vi "Quad PID 2015.vi"(0 "Target Velocity (rev/sec) 1":dbl, 1 "Measured Velocity (rev/sec) 1":dbl, 2 "Measured Velocity (rev/sec) 2":dbl, 3 "PID gains":T2 {"derivative time (Td, min)" format="%.3f"; "integral time (Ti, min)" format="%.3f"; "proportional gain (Kc)" format="%.3f"}, 5 "Target Velocity (rev/sec) 2":dbl, 9 "Target Velocity (rev/sec) 3":dbl, 11 "Target Velocity (rev/sec) 4":dbl, 12 "Measured Velocity (rev/sec) 3":dbl, 13 "Measured Velocity (rev/sec) 4":dbl, 14 "output range":cluster{"output high":dbl, "output low":dbl}={"output high"=1.0, "output low"=-1.0} {"output low" format="%.2f"; "output high" format="%.2f"}) -> (4 "Output Value (-1 to +1) 1":dbl format="%.2f", 6 "Output Value (-1 to +1) 2":dbl format="%.2f", 8 "Output Value (-1 to +1) 3":dbl format="%.2f", 10 "Output Value (-1 to +1) 4":dbl format="%.2f")   [LabVIEW 2014]
uses:
  <vilib>/Rock Robotics/WPI/DriverStation/WPI_DriverStationRobotMode2.ctl
  Robot Global Data.vi
  <vilib>/addons/control/pid/pid.llb/PID (DBL).vi
  <vilib>/addons/control/pid/NI_PID_pid.lvlib
panel:
  out "output cluster":T1(graph)
  in  "PID gains 2":T2={"proportional gain (Kc)"=2.0999999999999996, "integral time (Ti, min)"=0.004, "derivative time (Td, min)"=0.0} {"derivative time (Td, min)" format="%.3f"; "integral time (Ti, min)" min=0.0 step=0.001 format="%.3f"; "proportional gain (Kc)" step=0.05 format="%.3f"}
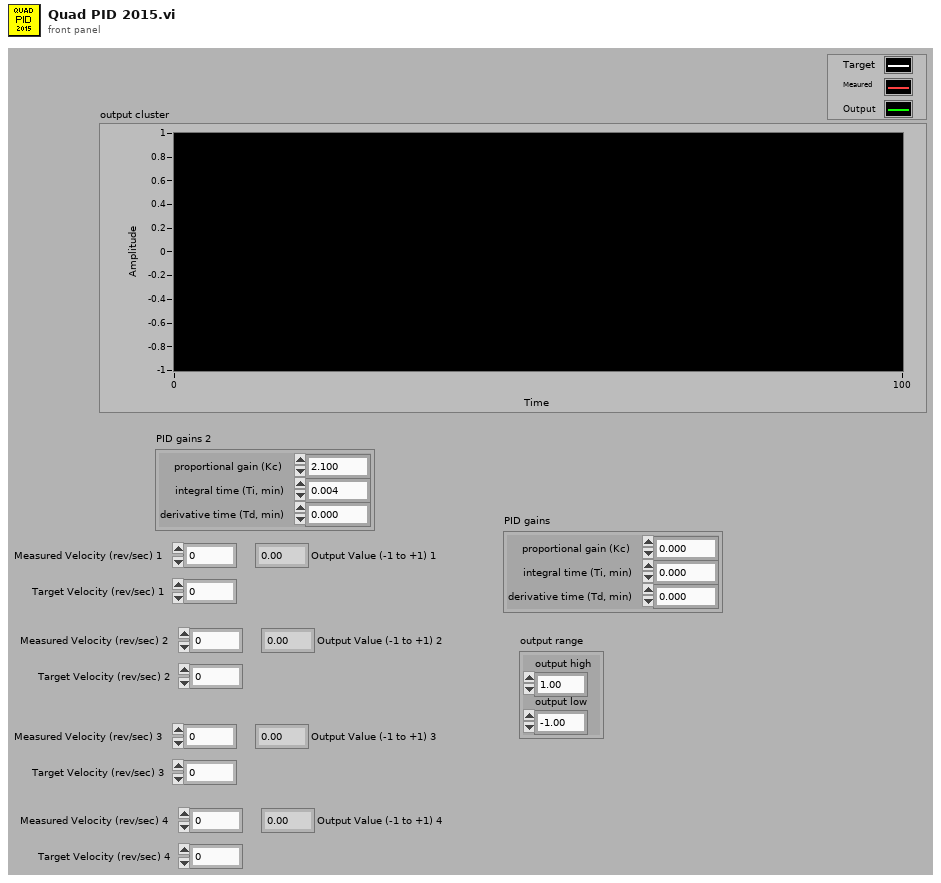
[diagram p1: front panel]
types:
  T1 = cluster{"Target Velocity (rev/sec) 1":dbl, "Measured Velocity (rev/sec) 1":dbl, "output":dbl}
  T2 = cluster{"proportional gain (Kc)":dbl, "integral time (Ti, min)":dbl, "derivative time (Td, min)":dbl}
  T3 = typedef "WPI_DriverStationRobotMode2.ctl" = enum16{"Autonomous Disabled", "Autonomous Enabled", "Teleop Disabled", "Teleop Enabled", "Disconnected", "Finish", "Test Disabled", "Test Enabled", "Emergency Stopped"}
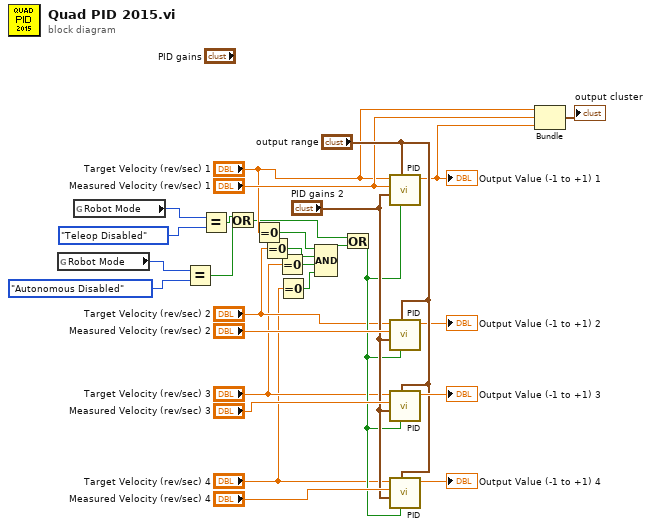
[diagram p0: block diagram]
diagram:
  n1 = global read "Robot Global Data.vi" "Robot Mode"() -> (w3:T3)
  n2 = global read "Robot Global Data.vi" "Robot Mode"() -> (w21:T3)
  n3 = Equal?(x=w3, y=WPI_DriverStationRobotMode2."Autonomous Disabled") -> (x = y?=w1:bool)
  n4 = Equal?(x=w21, y=WPI_DriverStationRobotMode2."Teleop Disabled") -> (x = y?=w5:bool)
  n5 = Or(x=w5, y=w1) -> (x .or. y?=w4:bool)
  n6 = Equal To 0?(x="Target Velocity (rev/sec) 1") -> (x = 0?=w9:bool)
  n7 = Equal To 0?(x="Target Velocity (rev/sec) 2") -> (x = 0?=w8:bool)
  n8 = Equal To 0?(x="Target Velocity (rev/sec) 3") -> (x = 0?=w7:bool)
  n9 = Equal To 0?(x="Target Velocity (rev/sec) 4") -> (x = 0?=w6:bool)
  n10 = Compound Arithmetic op=AND(w9, w8, w7, w6) -> (w14:bool)
  n11 = Or(x=w4, y=w14) -> (x .or. y?=w15:bool)
  n12 = call-poly <vilib>:"PID.vi"("reinitialize? (F)"=w15, "output range"="output range", "PID gains"="PID gains 2", "process variable"="Measured Velocity (rev/sec) 1", "setpoint"="Target Velocity (rev/sec) 1") -> ("output"=w16:dbl)  [unwired: 5 in, 1 out]
  "Output Value (-1 to +1) 1" <- w16
  n13 = call-poly <vilib>:"PID.vi"("reinitialize? (F)"=w15, "output range"="output range", "PID gains"="PID gains 2", "process variable"="Measured Velocity (rev/sec) 2", "setpoint"="Target Velocity (rev/sec) 2") -> ("output"=→"Output Value (-1 to +1) 2":dbl)  [unwired: 5 in, 1 out]
  n14 = call-poly <vilib>:"PID.vi"("reinitialize? (F)"=w15, "output range"="output range", "PID gains"="PID gains 2", "process variable"="Measured Velocity (rev/sec) 3", "setpoint"="Target Velocity (rev/sec) 3") -> ("output"=→"Output Value (-1 to +1) 3":dbl)  [unwired: 5 in, 1 out]
  n15 = call-poly <vilib>:"PID.vi"("reinitialize? (F)"=w15, "output range"="output range", "PID gains"="PID gains 2", "process variable"="Measured Velocity (rev/sec) 4", "setpoint"="Target Velocity (rev/sec) 4") -> ("output"=→"Output Value (-1 to +1) 4":dbl)  [unwired: 5 in, 1 out]
  n16 = Bundle("Target Velocity (rev/sec) 1"="Target Velocity (rev/sec) 1", "Measured Velocity (rev/sec) 1"="Measured Velocity (rev/sec) 1", "output"=w16) -> (→"output cluster":T1)  [unwired: 1 in]
